vi "Floating Messagebox.vi"(2 "Timeout":dbl[unit], 3 "Display Message":string) -> (0 "timed out":bool)   [LabVIEW 2015, in "CS++Utilities.lvlib"]
doc: "Display a message string in floating window for some time.\nUser can stop waiting by clicking in window or hitting <RETURN>-Key."
uses:
  CS++Utilities.lvlib
panel:
  out "Display Message":string
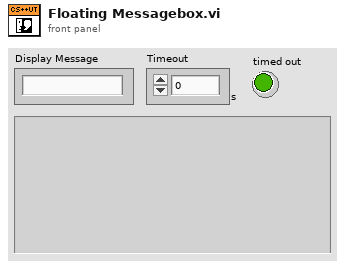
[diagram p1: front panel]
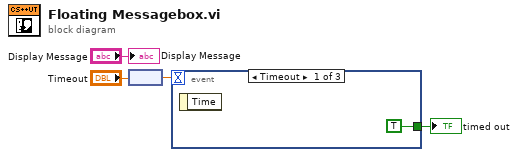
[diagram p0: block diagram]
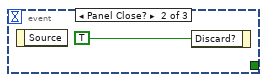
[diagram p2: hidden frame]
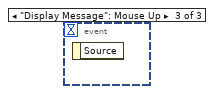
[diagram p3: hidden frame]
diagram:
  n1 = node("Timeout") -> (w3:dbl)
  n2 = event shown="[0] Timeout" {
    selector: _ -> [_ _ _]
    dyn-events: _ -> [_ _ _]
    timeout: w3 -> [_ _ _]
    tunnel: [TRUE _ _] -> w2
    event Timeout {
      n3 = event-data() -> ()  [unwired: 1 in, 1 out]
    }
    event Panel Close? {
      n4 = event-data() -> ()  [unwired: 1 in, 1 out]
      n5 = event-data("Discard?"=TRUE) -> ()  [unwired: 1 in, 1 out]
    }
    event "Display Message": Mouse Up {
      n6 = event-data() -> ()  [unwired: 1 in, 1 out]
    }
  }
  "timed out" <- w2
  "Display Message" <- "Display Message"
